vi "Get Nodes.vi"(8 "Error In":errorcluster, 11 "reference in":refnum<class "Network Mangement.lvclass">) -> (0 "Error Out":errorcluster, 2 "Nodes":map{u8, u8}(c390), 3 "reference out":refnum<class "Network Mangement.lvclass">)   [LabVIEW 2024, in "Network Mangement.lvclass"]
uses:
  Network Mangement.lvclass
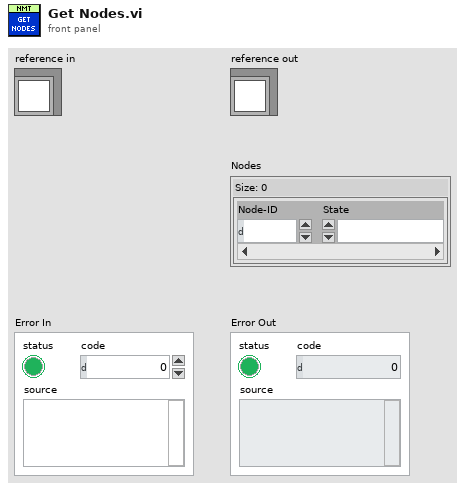
[diagram p1: front panel]
types:
  T1 = typedef "Network Mangement.lvclass/ObjectAttributes.ctl" = cluster{"Nodes":map{u8, u8}, "Heartbeats":map{u8, cluster{"Period":u16, "Timeout":u16, "Last Beat":timestamp}}, "Events":cluster{"Stop Heartbeat Checker":refnum<user-event>, "Heartbeat Timeout":refnum<user-event>, "Heartbeat Checker Error":refnum<user-event>}, "Heartbeat Checker":refnum<vi>}
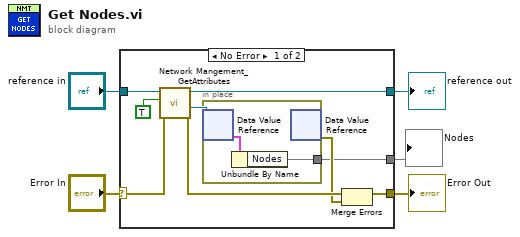
[diagram p0: block diagram]
diagram:
  n1 = case shown="No Error" "Error In" {
    selector: "Error In" -> [w14 w18]
    tunnel: [w12 w18] -> w4
    tunnel: [w9 w17] -> w2
    tunnel: "reference in" -> [w10 w17]
    tunnel: [w6 _] -> w1
    frame No Error {
      n2 = call "Network Mangement_GetAttributes.vi"("Error In"=w14, "OnlyGetDvrReference(False)"=TRUE, "reference in"=w10) -> ("Error Out"=w13:errorcluster, "DataRef"=w7:refnum<data-value>, "reference out"=w9:refnum<class "Network Mangement.lvclass">)  [unwired: 5 in, 1 out]
      n3 = in-place {
        in-place-border: [w16] -> w6
        n4 = in-place-dvr #1(w7) -> (w15:T1)  [unwired: 1 out]
        n5 = Unbundle By Name(w15) -> ("Nodes"=w16:map{u8, u8})
        n6 = in-place-dvr #1() -> (w11:errorcluster)  [unwired: 1 in, 1 out]
      }
      n7 = Merge Errors(w13, w11) -> (w12:errorcluster)
    }
    frame Error {
    }
  }
  "Error Out" <- w4
  "reference out" <- w2
  "Nodes" <- w1
